vi "tsfifo_delete_can_canfd_pass_filter.vi"(8 "error in (no error)":errorcluster caption="错误输入（无错误）", 9 "AIdentifier":i32, 10 "AIdxChn":i32, 11 "路径输入":path) -> (0 "error out":errorcluster caption="错误输出", 2 "function return":i32, 3 "路径输出":path)   [LabVIEW 2014]
doc: "Function Introduction :\nUnload CAN and CanFD messages through filters\nCall location :\ninput parameter :\nAChn: Channel :\nAIdentifier: Message ID\nReturn value :\n==0: Execution successful\nOther values: Query error code"
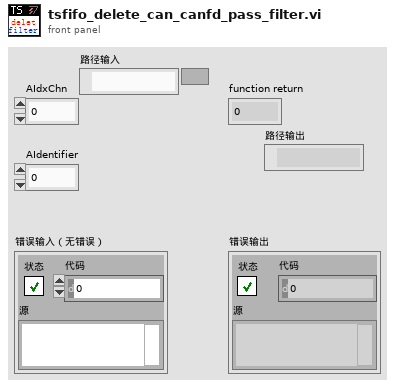
[diagram p1: front panel]
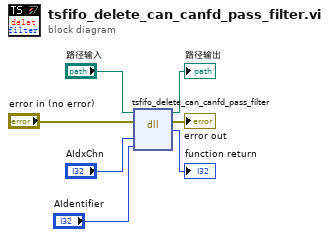
[diagram p0: block diagram]
diagram:
  n1 = dll-call lib="D:/Work/LabVIEW Code/TSMaster Labview SDK/LabVIEW/LabVIEW-TSMasterAPI_CLN/TSMasterAPI_LabVIEW-2024-08-30 15-02-46/Not_organized_vi/TSMaster.*" fn="tsfifo_delete_can_canfd_pass_filter"(path in="路径输入", error in="error in (no error)", "AIdxChn"="AIdxChn", "AIdentifier"="AIdentifier") -> (path out=→"路径输出":path, error out=→"error out":errorcluster, "返回类型"=→"function return":i32)  [unwired: 3 in]
